vi "FillArrByLinar.vi"(1 "Filling refence array":dbl[](array[numeric]), 2 "Cluster Array":cluster{dbl, dbl}[](array[cluster])) -> (0 "Filled Cluster Array":cluster{dbl, dbl}[](array[cluster]))   [LabVIEW 2016]
panel:
  # "This VI is to filling a cluster array with a \"standard\" array as filling reference.\nNOTE: Both cluster array and  \"standard\" array here must be ASC order sorted and has the same head(min,default is 0) and tail(max,default is 1) element .\n                \n             only a few of element are different.\n\nHow it works?\n\nwe define first element of cluster array as index,actullly it is a DBL value.and,define second element of cluster is var. \n\nif index of cluster array is equal to the  one of \"standard\" array's element. do nothing.\nelse insert into  a cluster to cluster array which index eqaul to \"standard\" array's element,and var is calcute by linar relation."
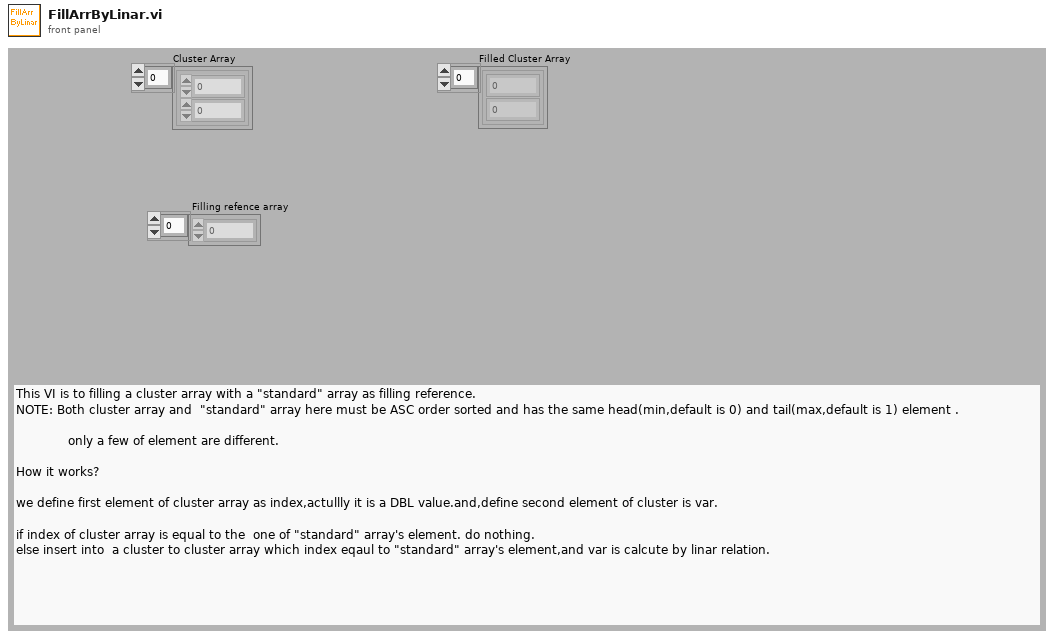
[diagram p1: front panel]
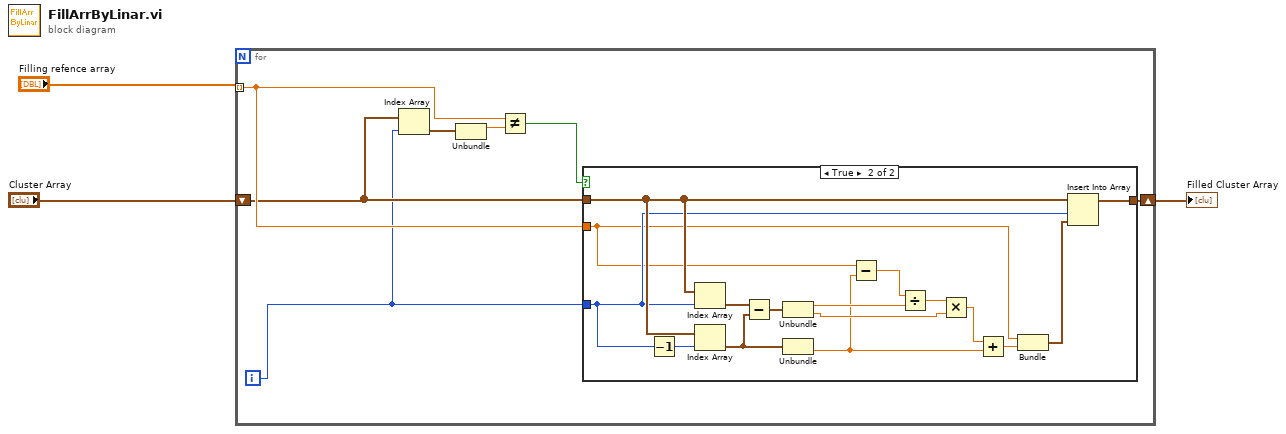
[diagram p0: block diagram]
diagram:
  n1 = for {
    tunnel: "Filling refence array" -> [w10] mode=indexing
    shift-right: [w9] -> w3
    shift-left: "Cluster Array" -> [w8]
    i -> [w4]
    n2 = Index Array(array=w8, index=w4) -> (element=w6:cluster{dbl, dbl})
    n3 = Unbundle(w6) -> (w5:dbl)  [unwired: 1 out]
    n4 = Not Equal?(x=w10, y=w5) -> (x != y?=w7:bool)
    n5 = case shown="True" w7 {
      tunnel: w8 -> [w11 w27]
      tunnel: w10 -> [_ w13]
      tunnel: w4 -> [_ w15]
      tunnel: [w11 w20] -> w9
      frame False {
      }
      frame True {
        n6 = Decrement(x=w15) -> (x-1=w14:i32)
        n7 = Index Array(array=w27, index=w15) -> (element=w26:cluster{dbl, dbl})
        n8 = Index Array(array=w27, index=w14) -> (element=w19:cluster{dbl, dbl})
        n9 = Subtract(x=w26, y=w19) -> (x-y=w25:cluster{dbl, dbl})
        n10 = Unbundle(w25) -> (w24:dbl, w22:dbl)
        n11 = Unbundle(w19) -> (w12:dbl)  [unwired: 1 out]
        n12 = Subtract(x=w13, y=w12) -> (x-y=w21:dbl)
        n13 = Divide(x=w21, y=w24) -> (x/y=w23:dbl)
        n14 = Multiply(x=w23, y=w22) -> (x*y=w18:dbl)
        n15 = Add(x=w18, y=w12) -> (x+y=w17:dbl)
        n16 = Bundle(w13, w17) -> (w16:cluster{dbl, dbl})  [unwired: 1 out]
        n17 = Insert Into Array(array=w27, index=w15, new element=w16) -> (w20:cluster{dbl, dbl}[])
      }
    }
  }
  "Filled Cluster Array" <- w3
